vi "lqManifestation.vi"(11 "LQIdentity in":refnum<class "LQIdentity.lvclass">) -> (2 "Manifestation":u64, 3 "LQIdentity out":refnum<class "LQIdentity.lvclass">)   [LabVIEW 2013, in "Template.lvlib" / "LQIdentity.lvclass"]
uses:
  LQIdentity.lvclass
  LQIdentity.lvclass/LQIdentity.ctl
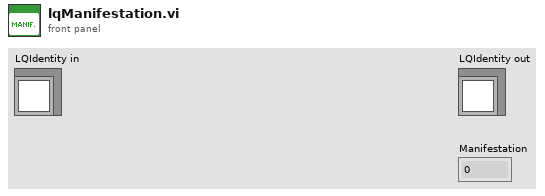
[diagram p1: front panel]
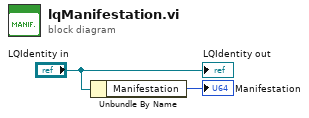
[diagram p0: block diagram]
diagram:
  n1 = Unbundle By Name("LQIdentity in") -> ("Manifestation"=→"Manifestation":u64)
  "LQIdentity out" <- "LQIdentity in"
